vi "Untitled 3.vi"() -> ()   [LabVIEW 2020]
uses:
  Control/State - Query Type.ctl
panel:
  out "resulting string":string
  in  "DATE_END":timestamp format="%<%d/%m/%Y>T"
  in  "DATE_START":timestamp format="%<%d/%m/%Y>T"
  out "Query String":string="SELECT `config_name`,`value` FROM `configuration` ORDER BY `id` ASC "
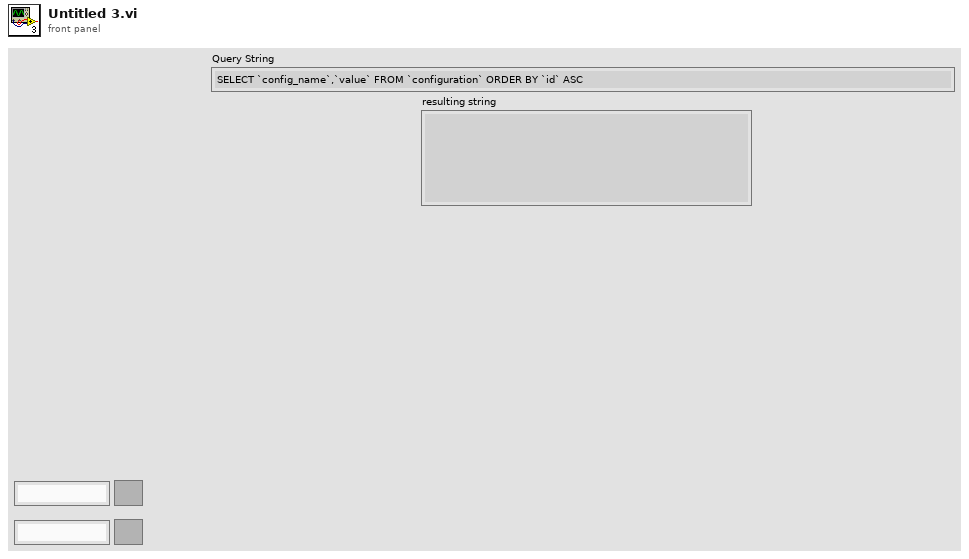
[diagram p1: front panel]
types:
  T1 = typedef "State - Query Type.ctl" = enum16{"SELECT", "UPDATE", "INSERT INTO", "TRUNCATE TABLE"}
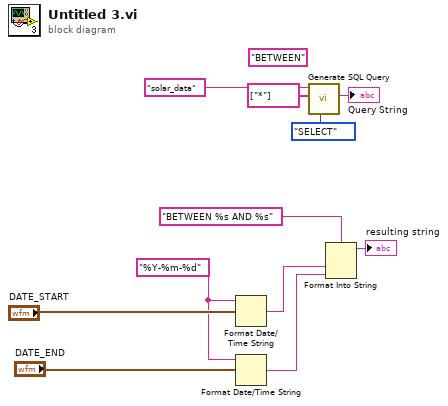
[diagram p0: block diagram]
diagram:
  w3 = "%Y-%m-%d" ("time format string (%c)")
  (unwired) "BETWEEN" ("Extra cmd")
  n1 = Format Date/Time String(time format string (%c)=w3, seconds (now)="DATE_START") -> (date/time string=w2:string)  [unwired: 1 in]
  n2 = Format Date/Time String(time format string (%c)=w3, seconds (now)="DATE_END") -> (date/time string=w1:string)  [unwired: 1 in]
  n3 = call "Generate SQL Query.vi"("Query type"=State_-_Query_Type."SELECT", "Column Name"=string[] ["*"], "Table Name"="solar_data") -> ("Query String"=→"Query String":string)  [unwired: 7 in, 1 out]
  n4 = Format Into String(format string="BETWEEN %s AND %s", w2, w1) -> (resulting string=→"resulting string":string)  [unwired: 2 in, 1 out]
